vi "Write Serialization.vi"(10 "Serialization":string, 11 "LQSerialData in":refnum<class "LQSerialData.lvclass">) -> (3 "LQSerialData out":refnum<class "LQSerialData.lvclass">)   [LabVIEW 2013, in "Template.lvlib" / "LQSerialData.lvclass"]
uses:
  LQSerialData.lvclass
  LQSerialData.lvclass/LQSerialData.ctl
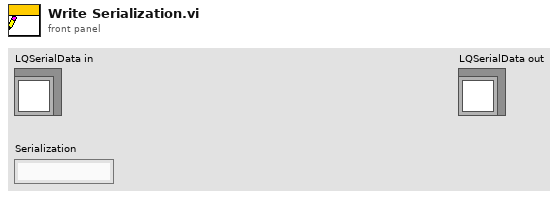
[diagram p1: front panel]
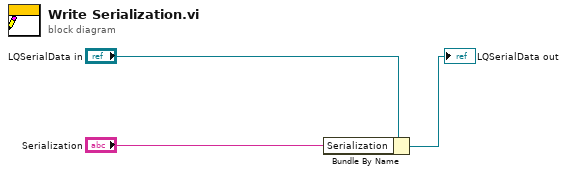
[diagram p0: block diagram]
diagram:
  n1 = Bundle By Name(cluster="LQSerialData in", "Serialization"="Serialization") -> (→"LQSerialData out":refnum<class "LQSerialData.lvclass">)
